vi "Thorlabs_CCS_Get_Device_Status.vi"(0 "VISA Refnum in":refnum<visa-resource-name>, 11 "error in (no error)":errorcluster) -> (4 "VISA Refnum out":refnum<visa-resource-name>, 6 "Scan is done":bool, 15 "error out":errorcluster)   [LabVIEW 2021]
doc: "This function retrieves whether the scan has run and is waiting for data to be transferred to the PC.\n\nThis function is a no blocking VI.\n\nAfter the 'Scan is done' indicator is true, the scan data can be read out with the 'Get Scan Data' function."
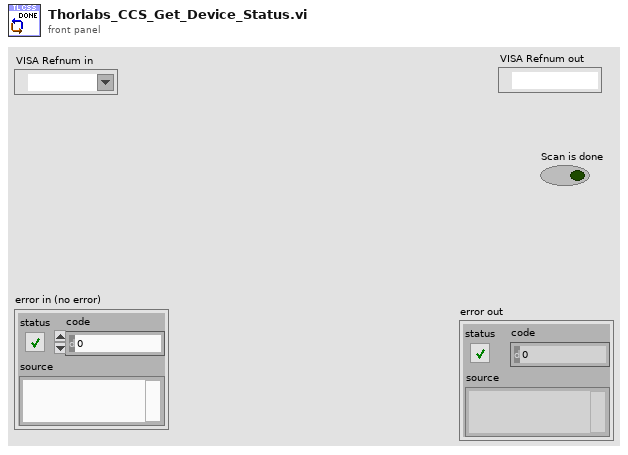
[diagram p1: front panel]
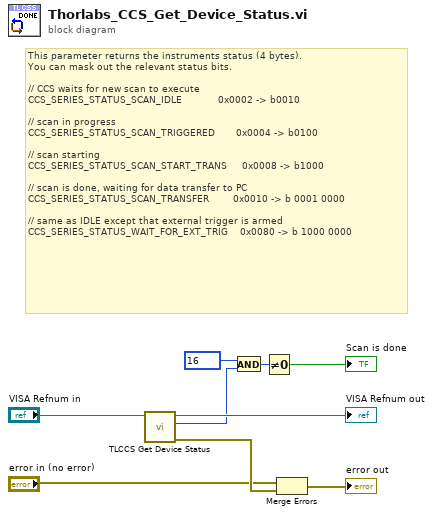
[diagram p0: block diagram]
diagram:
  # "This parameter returns the instruments status (4 bytes).\nYou can mask out the relevant status bits.\n\n// CCS waits for new scan to execute \nCCS_SERIES_STATUS_SCAN_IDLE            0x0002 -> b0010\n\n// scan in progress  \nCCS_SERIES_STATUS_SCAN_TRIGGERED       0x0004 -> b0100\n\n// scan starting  \nCCS_SERIES_STATUS_SCAN_START_TRANS     0x0008 -> b1000\n  \n// scan is done, waiting for data transfer to PC\nCCS_SERIES_STATUS_SCAN_TRANSFER        0x0010 -> b 0001 0000\n\n// same as IDLE except that external trigger is armed    \nCCS_SERIES_STATUS_WAIT_FOR_EXT_TRIG    0x0080 -> b 1000 0000"
  n1 = call <instrlib>:"TLCCS Get Device Status.vi"("instrument handle"="VISA Refnum in") -> ("error out"=w8:errorcluster, "Device Status"=w5:i32, "instrument handle out"=→"VISA Refnum out":refnum<visa-resource-name>)  [unwired: 8 in]
  n2 = And(x=16, y=w5) -> (x .and. y?=w1:i32)
  n3 = Not Equal To 0?(x=w1) -> (x != 0?=→"Scan is done":bool)
  n4 = Merge Errors("error in (no error)", w8) -> (→"error out":errorcluster)
